vi "XYGraphAddScaler.vi"(1 "y":dbl, 2 "XY Graph":cluster{"1D arrays":dbl[], dbl[]}[](array[cluster])) -> (0 "Array":cluster{"1D arrays":dbl[], dbl[]}[](array[cluster]))   [LabVIEW 2010]
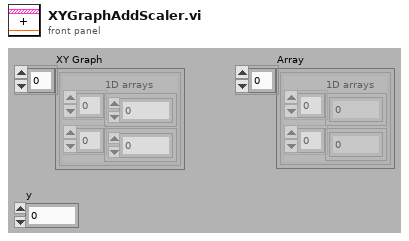
[diagram p1: front panel]
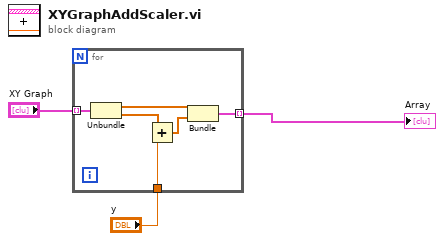
[diagram p0: block diagram]
diagram:
  n1 = for {
    tunnel: "XY Graph" -> [w9] mode=indexing
    tunnel: [w7] -> w2 mode=indexing
    tunnel: "y" -> [w4]
    n2 = Unbundle(w9) -> ("1D arrays"=w8:dbl[], w5:dbl[])
    n3 = Add(x=w5, y=w4) -> (x+y=w6:dbl[])
    n4 = Bundle("1D arrays"=w8, w6) -> (w7:cluster{"1D arrays":dbl[], dbl[]})  [unwired: 1 out]
  }
  "Array" <- w2
